vi "Shut_Down_Client_Demands.vi"(1 "Ch Names":string[](array[string]), 2 "Values":dbl[](array[numeric]) format="%.2f", 3 "Client Name":string) -> (0 "Comments":string)   [LabVIEW 2021]
uses:
  ADAM_Global.vi
  Anemometry/Anemometry Sub Vis/Globals/Constants_global.vi
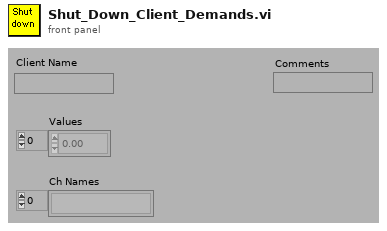
[diagram p1: front panel]
types:
  T1 = typedef "Server_Control.ctl" = cluster{"Channel Name to control":string, "Channel sharing":enum16{"Channel Unshared", "Channel Shared by Rig", "Channel Shared by Group"}, "Default Value":dbl, "Client Array":string[], "Time Stamp":timestamp, "Do Not Reset":bool}
  T2 = enum16{"Channel Unshared", "Channel Shared by Rig", "Channel Shared by Group"}
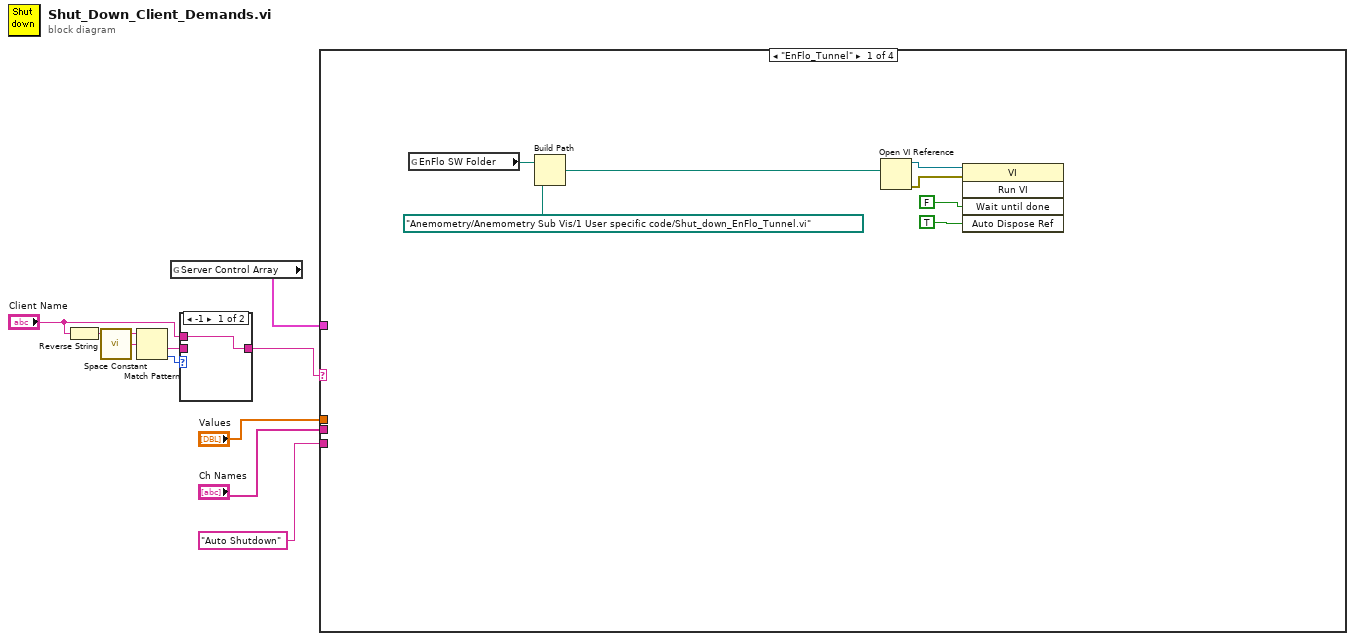
[diagram p0: block diagram]
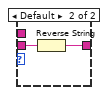
[diagram p2: hidden frame]
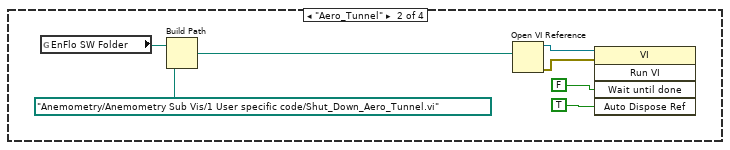
[diagram p3: hidden frame]
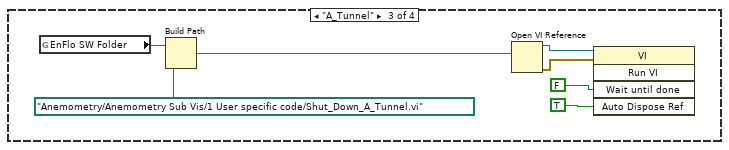
[diagram p4: hidden frame]
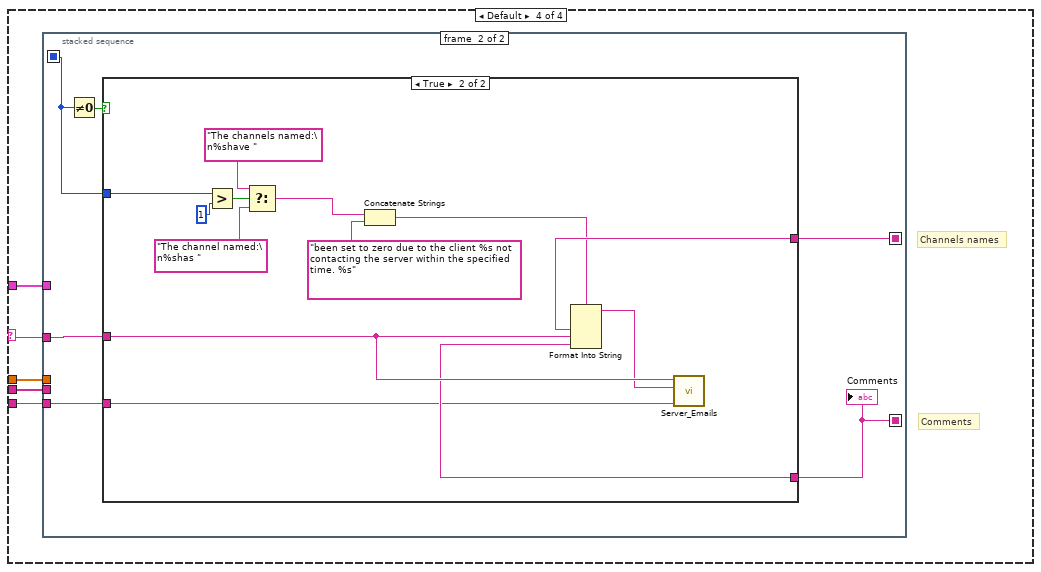
[diagram p5: hidden frame]
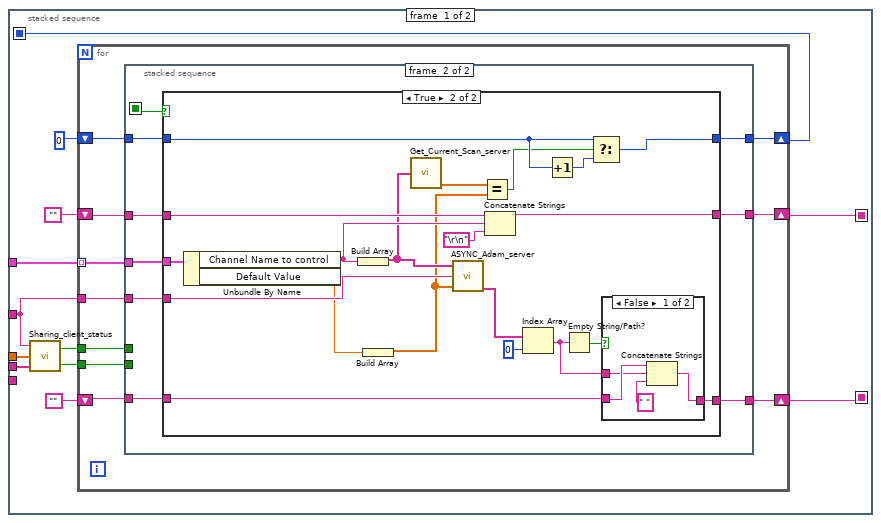
[diagram p6: hidden frame]
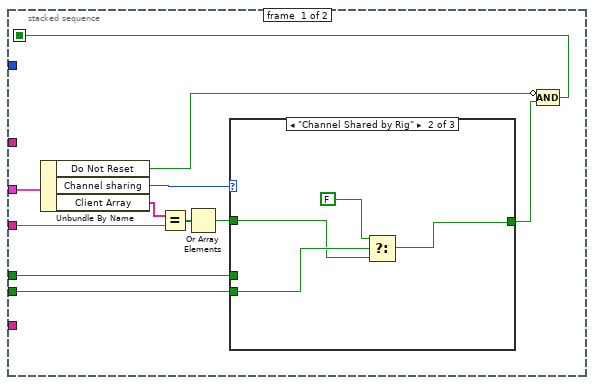
[diagram p7: hidden frame]
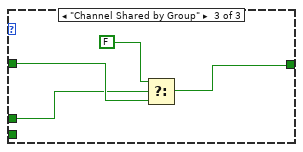
[diagram p9: hidden frame]
diagram:
  n1 = Reverse String(1:"Client Name") -> (0:w4:string)
  n2 = call <vilib>:"Space Constant.vi"() -> ("String"=w5:string)
  n3 = Match Pattern(string=w4, regular expression=w5) -> (after substring=w6:string, offset past match=w3:i32)  [unwired: 1 in, 2 out]
  n4 = global read "ADAM_Global.vi" "Server Control Array"() -> (w10:T1[])
  n5 = case shown="-1" w3 {
    tunnel: w6 -> [_ w13]
    tunnel: [w11 w12] -> w1
    tunnel: "Client Name" -> [w11 _]
    frame -1 {
    }
    frame Default {
      n6 = Reverse String(1:w13) -> (0:w12:string)
    }
  }
  n7 = case shown="\"EnFlo_Tunnel\"" w1 {
    selector: w1 -> [_ _ _ w35]
    tunnel: w10 -> [_ _ _ w39]
    tunnel: "Values" -> [_ _ _ w38]
    tunnel: "Ch Names" -> [_ _ _ w37]
    tunnel: "Auto Shutdown" ("Subject") -> [_ _ _ w36]
    frame "EnFlo_Tunnel" {
      n8 = global read "Constants_global.vi" "EnFlo SW Folder"() -> (w20:path)
      n9 = Build Path(base path=w20, name or relative path=path "Anemometry/Anemometry Sub Vis/1 User specific code/Shut_down_EnFlo_Tunnel.vi") -> (appended path=w14:path)
      n10 = Open VI Reference(vi path=w14) -> (vi reference=w16:refnum<vi>, error out=w15:errorcluster)  [unwired: 1 in, 4 out]
      n11 = invoke class="VI" method="Run VI"(reference=w16, error in=w15, "Wait until done"=FALSE, "Auto Dispose Ref"=TRUE) -> ()  [unwired: 1 in, 5 out]
    }
    frame "Aero_Tunnel" {
      n12 = global read "Constants_global.vi" "EnFlo SW Folder"() -> (w27:path)
      n13 = Build Path(base path=w27, name or relative path=path "Anemometry/Anemometry Sub Vis/1 User specific code/Shut_Down_Aero_Tunnel.vi") -> (appended path=w21:path)
      n14 = Open VI Reference(vi path=w21) -> (vi reference=w23:refnum<vi>, error out=w22:errorcluster)  [unwired: 1 in, 4 out]
      n15 = invoke class="VI" method="Run VI"(reference=w23, error in=w22, "Wait until done"=FALSE, "Auto Dispose Ref"=TRUE) -> ()  [unwired: 1 in, 5 out]
    }
    frame "A_Tunnel" {
      n16 = global read "Constants_global.vi" "EnFlo SW Folder"() -> (w34:path)
      n17 = Build Path(base path=w34, name or relative path=path "Anemometry/Anemometry Sub Vis/1 User specific code/Shut_Down_A_Tunnel.vi") -> (appended path=w28:path)
      n18 = Open VI Reference(vi path=w28) -> (vi reference=w30:refnum<vi>, error out=w29:errorcluster)  [unwired: 1 in, 4 out]
      n19 = invoke class="VI" method="Run VI"(reference=w30, error in=w29, "Wait until done"=FALSE, "Auto Dispose Ref"=TRUE) -> ()  [unwired: 1 in, 5 out]
    }
    frame Default {
      # "Channels names"
      # "Comments"
      n20 = stacked-sequence {
        seq-local: [w43 _] -> [_ w123]
        seq-local: [w44 _] -> [_ w120]
        seq-local: [w42 _] -> [_ w122]
        tunnel: w39 -> [w51 _]
        tunnel: w35 -> [w45 w121]
        tunnel: w38 -> [w41 _]
        tunnel: w37 -> [w40 _]
        tunnel: w36 -> [_ w119]
        frame #0 {
          n21 = call "Sharing_client_status.vi"("Ch Names"=w40, "Values"=w41, "Client Name"=w45) -> ("Active Machines in Rig"=w50:bool, "Active Machines in Group"=w49:bool)
          n22 = for {
            tunnel: w51 -> [w61] mode=indexing
            tunnel: w45 -> [w60]
            tunnel: w50 -> [w59]
            tunnel: w49 -> [w58]
            shift-right: [w56] -> w44
            shift-left: "" -> [w57]
            shift-right: [w54] -> w42
            shift-left: "" -> [w55]
            shift-right: [w52] -> w43
            shift-left: 0 -> [w53]
            n23 = stacked-sequence {
              seq-local: [w62 _] -> [_ w90]
              tunnel: w61 -> [w72 w89]
              tunnel: w60 -> [w69 w88]
              tunnel: w59 -> [w67 _]
              tunnel: w58 -> [w66 _]
              tunnel: w57 -> [_ w87]
              tunnel: [_ w86] -> w56
              tunnel: w55 -> [_ w85]
              tunnel: [_ w84] -> w54
              tunnel: w53 -> [_ w83]
              tunnel: [_ w82] -> w52
              frame #0 {
                n24 = Unbundle By Name(w72) -> ("Do Not Reset"=w63:bool, "Channel sharing"=w71:T2, "Client Array"=w70:string[])
                n25 = Equal?(x=w70, y=w69) -> (x = y?=w68:bool[])
                n26 = Or Array Elements(Boolean array=w68) -> (logical OR=w65:bool)
                n27 = case shown="\"Channel Shared by Rig\"" w71 {
                  tunnel: [w73 w74 w79] -> w64
                  tunnel: w65 -> [w73 w76 w81]
                  tunnel: w67 -> [_ w77 _]
                  tunnel: w66 -> [_ _ w78]
                  frame "Channel Unshared" {
                  }
                  frame "Channel Shared by Rig" {
                    n28 = Select(t=FALSE, s=w77, f=w76) -> (s? t:f=w74:bool)
                  }
                  frame "Channel Shared by Group" {
                    n29 = Select(t=FALSE, s=w78, f=w81) -> (s? t:f=w79:bool)
                  }
                }
                n30 = Compound Arithmetic op=AND(invert w63, w64) -> (w62:bool)
              }
              frame #1 {
                n31 = case shown="True" w90 {
                  tunnel: w89 -> [_ w113]
                  tunnel: w88 -> [_ w106]
                  tunnel: w87 -> [w93 w110]
                  tunnel: [w93 w109] -> w86
                  tunnel: w85 -> [w91 w105]
                  tunnel: [w91 w104] -> w84
                  tunnel: w83 -> [w92 w97]
                  tunnel: [w92 w98] -> w82
                  frame False {
                  }
                  frame True {
                    n32 = Unbundle By Name(w113) -> ("Channel Name to control"=w103:string, "Default Value"=w102:dbl)
                    n33 = Build Array(w103) -> (w101:string[])
                    n34 = Build Array(w102) -> (w99:dbl[])
                    n35 = call "Get_Current_Scan_server.vi"("Desired Channels"=w101) -> ("Numerical Values"=w100:dbl[])  [unwired: 2 out]
                    n36 = call "ASYNC_Adam_server.vi"("Values"=w99, "Client Name"=w106, "Channel Names"=w101) -> ("Scan Comments"=w112:string[])  [unwired: 2 out]
                    n37 = Equal?(x=w100, y=w99) -> (x = y?=w95:bool)
                    n38 = Concatenate Strings(w105, w103, "\r\n") -> (w104:string)
                    n39 = Index Array(array=w112, index=0 ("Index")) -> (element=w107:string)
                    n40 = Increment(x=w97) -> (x+1=w96:i32)
                    n41 = Empty String/Path?(string/path=w107) -> (empty?=w108:bool)
                    n42 = Select(t=w97, s=w95, f=w96) -> (s? t:f=w98:i32)
                    n43 = case shown="False" w108 {
                      tunnel: w110 -> [w116 w118]
                      tunnel: [w117 w118] -> w109
                      tunnel: w107 -> [w115 _]
                      frame False {
                        n44 = Concatenate Strings(w116, w115, " ") -> (w117:string)
                      }
                      frame True {
                      }
                    }
                  }
                }
              }
            }
          }
        }
        frame #1 {
          n45 = Not Equal To 0?(x=w123) -> (x != 0?=w124:bool)
          n46 = case shown="True" w124 {
            tunnel: w123 -> [_ w137]
            tunnel: w122 -> [_ w136]
            tunnel: w121 -> [_ w135]
            tunnel: w120 -> [_ w134]
            tunnel: w119 -> [_ w125]
            frame False {
            }
            frame True {
              n47 = Greater?(x=w137, y=1) -> (0:w131:bool)
              n48 = Select(t="The channels named:\n%shave ", s=w131, f="The channel named:\n%shas ") -> (s? t:f=w129:string)
              n49 = Concatenate Strings(w129, "been set to zero due to the client %s not contacting the server within the specified time. %s" ("Substring")) -> (w127:string)
              n50 = Format Into String(format string=w127, w136, w135, w134) -> (resulting string=w126:string)  [unwired: 2 in, 1 out]
              n51 = call "Server_Emails.vi"("Client Name Contains"=w135, "Message"=w126, "Subject"=w125) -> ()  [unwired: 2 in, 3 out]
            }
          }
          "Comments" <- w120
        }
      }
    }
  }
